vi "Create.vi"(8 "error in (no error)":errorcluster, 9 "Length":u64=1, 10 "From":u64) -> (0 "error out":errorcluster, 3 "Range":refnum<class "Range.lvclass">)   [LabVIEW 2020, in "Range.lvclass"]
uses:
  Range.lvclass
  Range.lvclass/Range.ctl
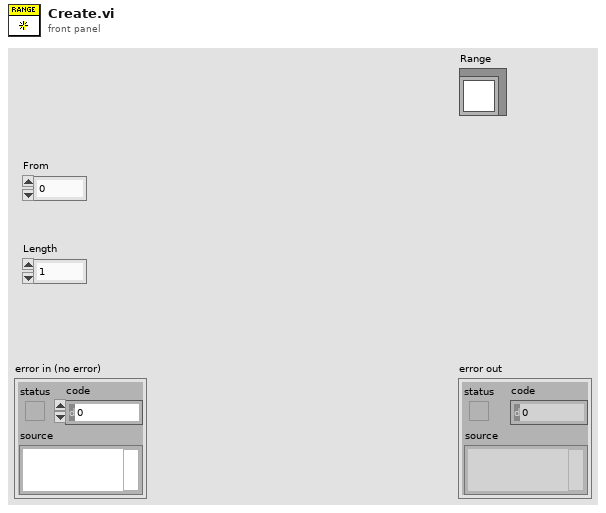
[diagram p1: front panel]
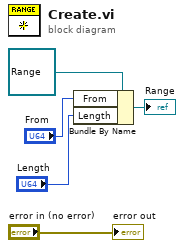
[diagram p0: block diagram]
diagram:
  n1 = Bundle By Name(cluster=refnum<class "Range.lvclass"> refnum ("Range"), "From"="From", "Length"="Length") -> (→"Range":refnum<class "Range.lvclass">)
  "error out" <- "error in (no error)"
